vi "S2C_XML_UpdateEventStatus.vi"(8 "Error In":errorcluster, 11 "Value":string) -> (0 "Error Out":errorcluster)   [LabVIEW 2015]
uses:
  S2C_XML_Globals.vi
  <vilib>/xml/Close Reference(Node).vi
  <resource>/objmgr/DOMUserDefRef.rc
  <vilib>/xml/NI_XML.lvlib
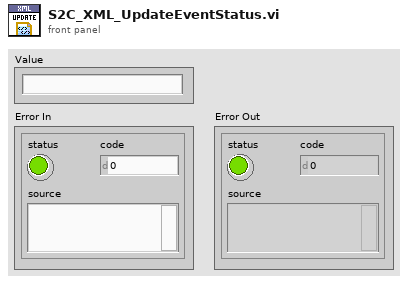
[diagram p1: front panel]
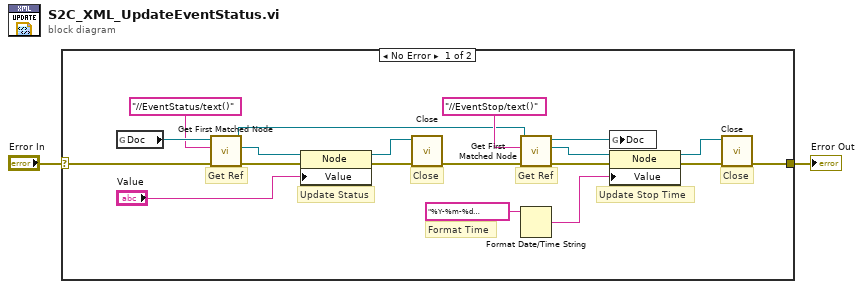
[diagram p0: block diagram]
diagram:
  n1 = case shown="No Error" "Error In" {
    selector: "Error In" -> [w17 w21]
    tunnel: [w20 w21] -> w2
    frame No Error {
      # "Format Time"
      # "Update Stop Time"
      # "Close"
      # "Get Ref"
      # "Update Status"
      # "Close"
      # "Get Ref"
      n2 = global read "S2C_XML_Globals.vi" "Doc"() -> (w19:refnum<k20>)
      n3 = call <vilib>:"Get First Matched Node.vi"("error in (no error)"=w17, "XPath expression"="//EventStatus/text()", "node in"=w19) -> ("error out"=w18:errorcluster, "node result"=w16:refnum<k20>, "node out"=w5:refnum<k20>)  [unwired: 6 in]
      n4 = property class="Node"(reference=w16, error in=w18, "Value"="Value") -> (reference out=w13:refnum<k20>, error out=w14:errorcluster)
      n5 = call-poly <vilib>:"Close.vi"("error in (no error)"=w14, "node"=w13) -> ("error out"=w20:errorcluster)  [unwired: 7 in]
      n6 = call <vilib>:"Get First Matched Node.vi"("XPath expression"="//EventStop/text()", "node in"=w5) -> ("error out"=w6:errorcluster, "node result"=w7:refnum<k20>, "node out"=w8:refnum<k20>)  [unwired: 7 in]
      n7 = Format Date/Time String(time format string (%c)="%Y-%m-%d %H:%M:%S%3u") -> (date/time string=w3:string)  [unwired: 2 in]
      n8 = global write "S2C_XML_Globals.vi" "Doc"(w8) -> ()
      n9 = property class="Node"(reference=w7, error in=w6, "Value"=w3) -> (reference out=w10:refnum<k20>, error out=w9:errorcluster)
      n10 = call-poly <vilib>:"Close.vi"("error in (no error)"=w9, "node"=w10) -> ()  [unwired: 7 in, 1 out]
    }
    frame Error {
    }
  }
  "Error Out" <- w2
